vi "RW_LiveVIew.vi"(9 "Task":enum16{"Read", "Write", "Init"}(ring), 11 "Plots":refnum<vi>[](array[refnum])) -> ()   [LabVIEW 2022 SP3]
uses:
  <vilib>/Utility/miscctls.llb/LVRangeTypeDef.ctl
panel:
  out "Data":T1[][](array[typedef])
  out "Pref Path":path
  out "File Out":string
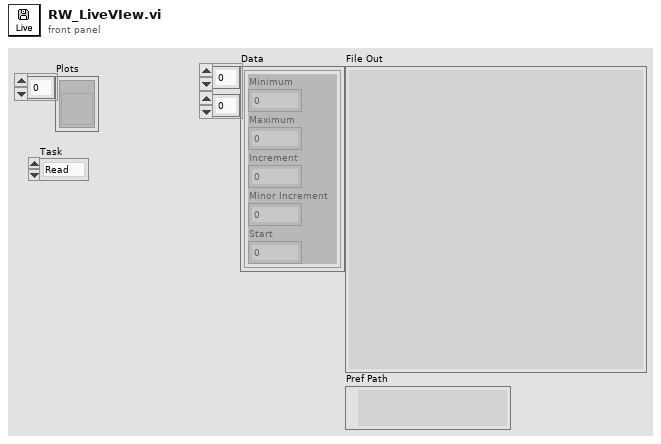
[diagram p1: front panel]
types:
  T1 = typedef "LVRangeTypeDef.ctl" = cluster{"Minimum":dbl, "Maximum":dbl, "Increment":dbl, "Minor Increment":dbl, "Start":dbl}
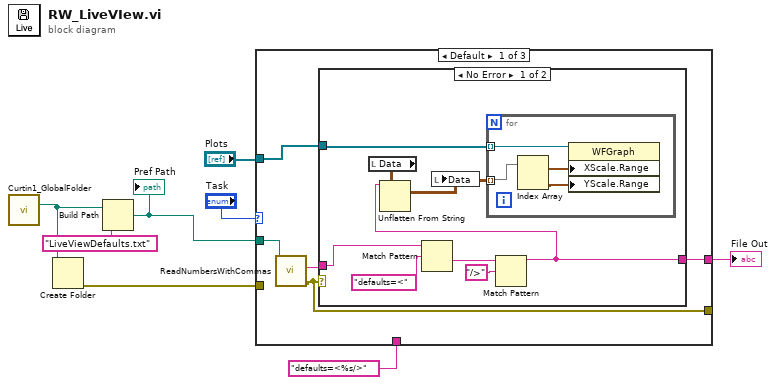
[diagram p0: block diagram]
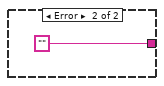
[diagram p2: hidden frame]
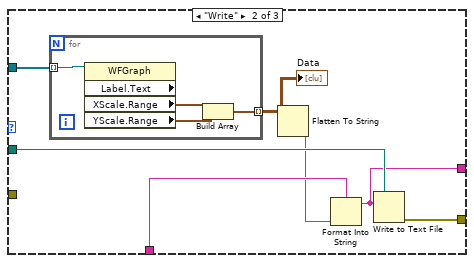
[diagram p3: hidden frame]
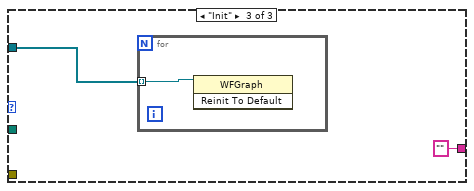
[diagram p4: hidden frame]
diagram:
  n1 = call "Curtin1_GlobalFolder.vi"() -> ("LabVIEW Data Path"=w4:path)  [unwired: 1 in, 1 out]
  n2 = Create Folder(path (use dialog)=w4) -> (error out=w5:errorcluster)  [unwired: 2 in, 2 out]
  n3 = Build Path(base path=w4, name or relative path="LiveViewDefaults.txt") -> (appended path=w8:path)
  "Pref Path" <- w8
  n4 = case shown="Default" "Task" {
    tunnel: w8 -> [w13 w33 _]
    tunnel: [w11 w32 _] -> _
    tunnel: [w10 w27 "" ("Notes")] -> w6
    tunnel: w5 -> [_ _ _]
    tunnel: "defaults=<%s/>" ("format string") -> [_ w31 _]
    tunnel: "Plots" -> [w9 w30 w39]
    frame Default {
      n5 = call "ReadNumbersWithCommas.vi"("file (use dialog)"=w13) -> ("error out"=w11:errorcluster, "text"=w12:string)  [unwired: 7 in, 2 out]
      n6 = case shown="No Error" w11 {
        tunnel: [w14 "" ("Notes")] -> w10
        tunnel: w12 -> [w21 _]
        tunnel: w9 -> [w16 _]
        frame No Error {
          n7 = local read "Data"() -> (w17:T1[][])
          n8 = Match Pattern(string=w21, regular expression="defaults=<" ("format string")) -> (after substring=w20:string)  [unwired: 1 in, 3 out]
          n9 = Match Pattern(string=w20, regular expression="/>" ("format string")) -> (before substring=w14:string)  [unwired: 1 in, 3 out]
          n10 = Unflatten From String(type=w17, binary string=w14) -> (value=w15:T1[][])  [unwired: 3 in, 2 out]
          n11 = local write "Data"(w15) -> ()
          n12 = for {
            tunnel: w16 -> [w25] mode=indexing
            tunnel: w15 -> [w24] mode=indexing
            n13 = Index Array(array=w24) -> (element #1=w23:T1, element #2=w22:T1)  [unwired: 2 in]
            n14 = property on="Property Node" class="WFGraph"(reference=w25, "XScale.Range"=w23, "YScale.Range"=w22) -> ()  [unwired: 1 in, 2 out]
          }
        }
        frame Error {
        }
      }
    }
    frame "Write" {
      n15 = for {
        tunnel: w30 -> [w37] mode=indexing
        tunnel: [w34] -> w29 mode=indexing
        n16 = property on="Property Node" class="WFGraph" props=["Label", "Text", "XScale", "Range", "YScale", "Range"](reference=w37) -> ("XScale.Range"=w36:T1, "YScale.Range"=w35:T1)  [unwired: 1 in, 3 out]
        n17 = Build Array(w36, w35) -> (w34:T1[])
      }
      "Data" <- w29
      n18 = Flatten To String(anything=w29) -> (data string=w28:string)  [unwired: 3 in, 2 out]
      n19 = Format Into String(format string=w31, w28) -> (resulting string=w27:string)  [unwired: 2 in, 1 out]
      n20 = Write to Text File(file (use dialog)=w33, text=w27) -> (error out=w32:errorcluster)  [unwired: 2 in, 2 out]
    }
    frame "Init" {
      n21 = for {
        tunnel: w39 -> [w40] mode=indexing
        n22 = invoke on="Invoke Node" class="WFGraph" method="Reinit To Default"(reference=w40) -> ()  [unwired: 2 in, 3 out]
      }
    }
  }
  "File Out" <- w6
